vi "Disconnect Channels (Single).vi"(8 "error in (no error)":errorcluster, 9 "channel 2":string, 10 "channel 1":string, 11 "SLSC Switch in":refnum<class "SLSC Switch.lvclass">) -> (0 "error out":errorcluster, 3 "SLSC Switch out":refnum<class "SLSC Switch.lvclass">)   [LabVIEW 2015, in "SLSC Switch.lvlib" / "SLSC Switch.lvclass"]
doc: "Breaks the path between two channels created with the Connect Channels VI. If no connection exists between the channels, SLSC-SWITCH returns an error."
uses:
  SLSC Switch.lvclass
  slscsl/slscsl.lvclass
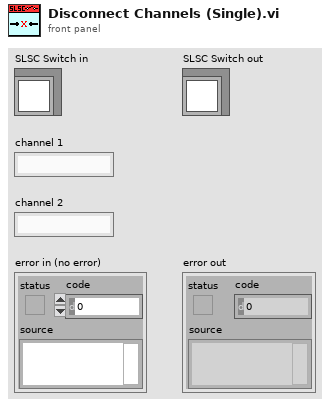
[diagram p1: front panel]
types:
  T1 = typedef "SLSC Switch.lvlib/slscsl.lvclass/SwitchActionsArray.ctl" = T2[]
  T2 = typedef "SLSC Switch.lvlib/slscsl.lvclass/SwitchAction.ctl" = cluster{"index":i32, "RelayAction":T3}
  T3 = typedef "SLSC Switch.lvlib/slscsl.lvclass/RelayAction.ctl" = u32
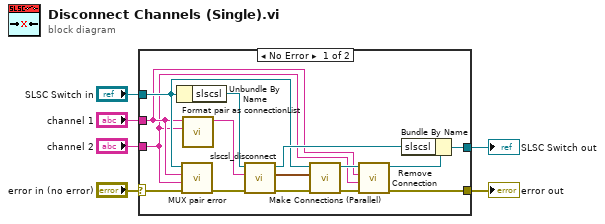
[diagram p0: block diagram]
diagram:
  n1 = case shown="No Error" "error in (no error)" {
    selector: "error in (no error)" -> [w8 w23]
    tunnel: [w21 w23] -> w5
    tunnel: "channel 1" -> [w10 _]
    tunnel: "channel 2" -> [w9 _]
    tunnel: [w20 w22] -> w2
    tunnel: "SLSC Switch in" -> [w11 w22]
    frame No Error {
      n2 = Unbundle By Name(w11) -> ("slscsl"=w19:refnum<class "slscsl.lvclass">)
      n3 = call "MUX pair error.vi"("error in (no error)"=w8, "channel 2"=w9, "channel 1"=w10, "SLSC Switch in"=w11) -> ("error out"=w7:errorcluster)  [unwired: 7 in]
      n4 = call "Format pair as connectionList.vi"("channel in"=w9, "channel 1"=w10) -> ("connectionList"=w16:string)  [unwired: 9 in]
      n5 = call "slscsl_disconnect.vi"("error in (no error)"=w7, "connectionList"=w16, "slscsl in"=w19) -> ("error out"=w17:errorcluster, "SwitchActionsArray"=w18:T1, "slscsl out"=w12:refnum<class "slscsl.lvclass">)  [unwired: 6 in]
      n6 = call "Make Connections (Parallel).vi"("error in (no error)"=w17, "switchActionsArray"=w18, "SLSC Switch in"=w11) -> ("error out"=w15:errorcluster, "SLSC Switch out"=w13:refnum<class "SLSC Switch.lvclass">)  [unwired: 7 in]
      n7 = call "Remove Connection.vi"("error in (no error)"=w15, "channel 2"=w9, "channel 1"=w10, "SLSC Switch in"=w13) -> ("error out"=w21:errorcluster, "SLSC Switch out"=w14:refnum<class "SLSC Switch.lvclass">)  [unwired: 6 in]
      n8 = Bundle By Name(cluster=w14, "slscsl"=w12) -> (w20:refnum<class "SLSC Switch.lvclass">)
    }
    frame Error {
    }
  }
  "error out" <- w5
  "SLSC Switch out" <- w2
